vi "1过0比较法子程序.vi"(1 "波形":waveform(dbl)) -> (0 "f":dbl)   [LabVIEW 2017]
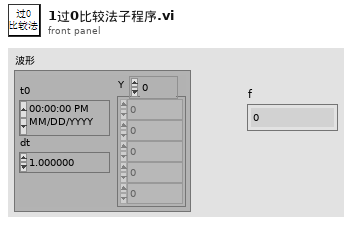
[diagram p1: front panel]
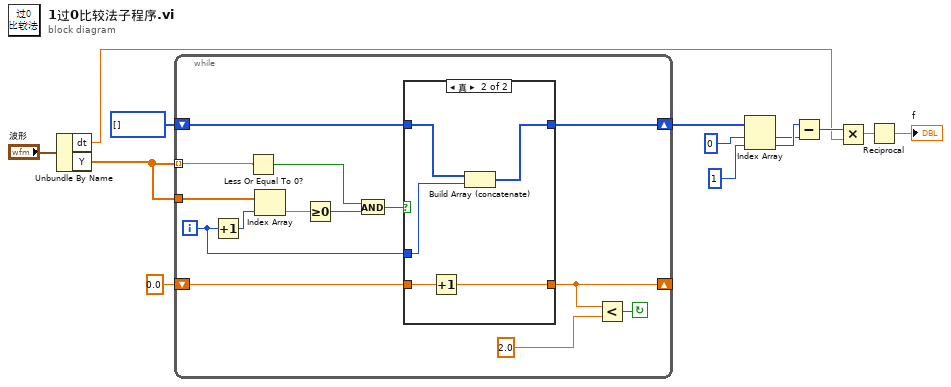
[diagram p0: block diagram]
diagram:
  n1 = Unbundle By Name("波形") -> ("dt"=w1:dbl, "Y"=w11:dbl[])
  n2 = while {
    tunnel: w11 -> [w24] mode=indexing
    tunnel: w11 -> [w27]
    shift-right: [w19] -> w8
    shift-left: i32[] [] -> [w20]
    shift-right: [w17] -> _
    shift-left: 0.0 -> [w18]
    i -> [w21]
    stop <- w15 continue-if-true
    n3 = Increment(x=w21) -> (x+1=w26:i32)
    n4 = Less Or Equal To 0?(x=w24) -> (x <= 0?=w22:bool)
    n5 = Index Array(array=w27, index=w26) -> (element=w25:dbl)
    n6 = Greater Or Equal To 0?(x=w25) -> (x >= 0?=w23:bool)
    n7 = And(x=w22, y=w23) -> (x .and. y?=w14:bool)
    n8 = case shown="真" w14 {
      tunnel: w21 -> [_ w34]
      tunnel: w20 -> [w29 w32]
      tunnel: [w29 w33] -> w19
      tunnel: w18 -> [w28 w31]
      tunnel: [w28 w30] -> w17
      frame False {
      }
      frame True {
        n9 = Increment(x=w31) -> (x+1=w30:dbl)
        n10 = Build Array (concatenate)(w32, w34) -> (w33:i32[])
      }
    }
    n11 = Less?(x=w17, y=2.0) -> (x < y?=w15:bool)
  }
  n12 = Index Array(array=w8, index #1=0 ("索引"), index #2=1 ("索引")) -> (element #1=w4:i32, element #2=w5:i32)
  n13 = Subtract(x=w5, y=w4) -> (x-y=w3:i32)
  n14 = Multiply(x=w3, y=w1) -> (x*y=w2:dbl)
  n15 = Reciprocal(x=w2) -> (1/x=→"f":dbl)
